vi "PID_VI.vi"(6 "Lock All":bool, 9 "millisecond multiple":u32, 10 "Single sensor PID parameters":T1(array[cluster]), 11 "Waveform":waveform(dbl)) -> (1 "laser setpoint":dbl[](array[numeric]), 2 "PD setpoint":dbl[](array[numeric]), 3 "data average":dbl[](array[numeric]))   [LabVIEW 2015]
uses:
  <vilib>/addons/control/pid/NI_PID_pid.lvlib
  <vilib>/addons/control/pid/pid.llb/PID (DBL).vi
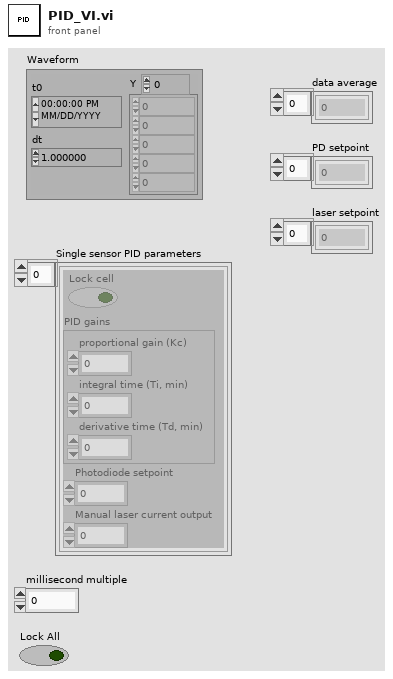
[diagram p1: front panel]
types:
  T1 = cluster{"Lock cell":bool, "PID gains":cluster{"proportional gain (Kc)":dbl, "integral time (Ti, min)":dbl, "derivative time (Td, min)":dbl}, "Photodiode setpoint":dbl, "Manual laser current output":dbl}[]
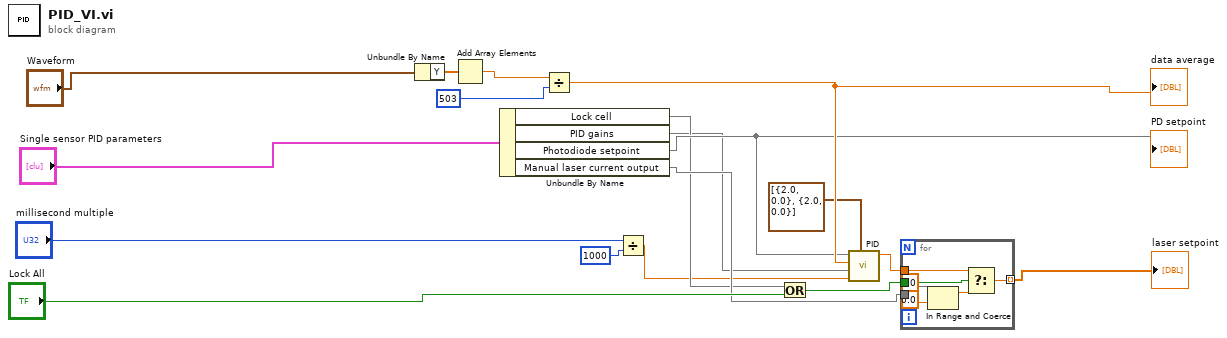
[diagram p0: block diagram]
diagram:
  n1 = Unbundle By Name("Waveform") -> ("Y"=w4:dbl[])
  n2 = Add Array Elements(numeric array=w4) -> (sum=w5:dbl)
  n3 = Unbundle By Name("Single sensor PID parameters") -> ("Lock cell"=w11, "PID gains"=w8, "Photodiode setpoint"=w17, "Manual laser current output"=w14)
  "PD setpoint" <- w17
  n4 = Divide(x=w5, y=503 ("samples per channel")) -> (x/y=w18:dbl)
  "data average" <- w18
  n5 = Divide(x="millisecond multiple", y=u32 1000) -> (x/y=w10:dbl)
  n6 = Or(x=w11, y="Lock All") -> (x .or. y?=w12:bool)
  n7 = call-poly <vilib>:"PID.vi"("output range"=cluster{"output high":dbl, "output low":dbl}[] [{"output high"=2.0, "output low"=0.0}, {"output high"=2.0, "output low"=0.0}], "dt (s)"=w10, "PID gains"=w8, "process variable"=w18, "setpoint"=w17) -> ("output"=w13:dbl)  [unwired: 5 in, 1 out]
  n8 = for {
    tunnel: w12 -> [w25]
    tunnel: w13 -> [w24]
    tunnel: w14 -> [w22]
    tunnel: [w23] -> w16 mode=indexing
    n9 = In Range and Coerce(upper limit=2.0, x=w22, lower limit=0.0) -> (coerced(x)=w21:dbl)  [unwired: 1 out]
    n10 = Select(t=w24, s=w25, f=w21) -> (s? t:f=w23:dbl)
  }
  "laser setpoint" <- w16
